vi "Check Board Status.vi"(8 "error in":errorcluster) -> (0 "error out":errorcluster, 3 "Ready?":bool)   [LabVIEW 2014]
uses:
  CAN Communication/PAS/PAS.lvclass
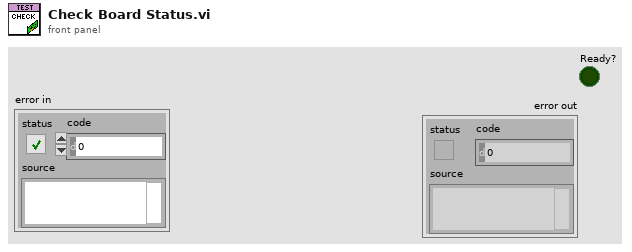
[diagram p1: front panel]
types:
  T1 = typedef "PAS.lvclass/Session Handle.ctl" = refnum<data-value>
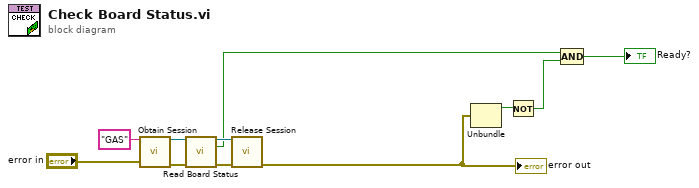
[diagram p0: block diagram]
diagram:
  n1 = call "Obtain Session.vi"("Session  Name ()"="GAS", "error in (no error)"="error in") -> ("Session Handle"=w9:T1, "error out"=w10:errorcluster)  [unwired: 12 in]
  n2 = call "Read Board Status.vi"("Session Handle in"=w9, "error in (no error)"=w10) -> ("Session Handle out"=w7:T1, "Ready?"=w5:bool, "error out"=w8:errorcluster)  [unwired: 11 in]
  n3 = call "Release Session.vi"("Session Handle"=w7, "error in (no error)"=w8) -> ("error out"=w1:errorcluster)  [unwired: 13 in]
  "error out" <- w1
  n4 = Unbundle(w1) -> ("status"=w4:bool)  [unwired: 2 out]
  n5 = Not(x=w4) -> (.not. x?=w3:bool)
  n6 = Compound Arithmetic op=AND(w5, w3) -> (→"Ready?":bool)
